vi "Edit_Template_File.vi"(0 "Mode":T2(ring), 7 "Template Filename":path, 11 "Data Filename":path) -> (6 "Template Filename Out":path)   [LabVIEW 2015]
uses:
  Anemometry/Anemometry Sub Vis/Data_plotting_vis/File_Template_Clus.ctl
  Anemometry/Anemometry Sub Vis/Controls/Global_mode.ctl
panel:
  out "index of element":i32
  in  "Add New Channel Named":bool
  in  "Edit Maths Equation":bool
  out "Current Case Name":string
  in  "Organise Channels":bool
  in  "Add New Channels Fr File":bool
  in  "OK":bool
  in  "Search String":string
  in  "Listbox":i32(listbox)
  out "Channel Name":string
  in  "Cluster":T1 {"Tolerance" min=0.0 format="%#.4f"}
  # "> 20  or  <20  or  =hello   or \n£hello  (not equal to hello)"
  # "<<Characters_to_Match>>  <<Replace_Whole_String_with_this>>"
  # "<<Channel_Name>> contains <<Characters to match>> or\n<<Channel_Name>> does not contain <<Characters to match>>"
  # "<<Channel_Name_A>> + <<Channel_Name_B>> or\nConcatenate <<Channel_Name_A>> and <<Channel_Name_B>>"
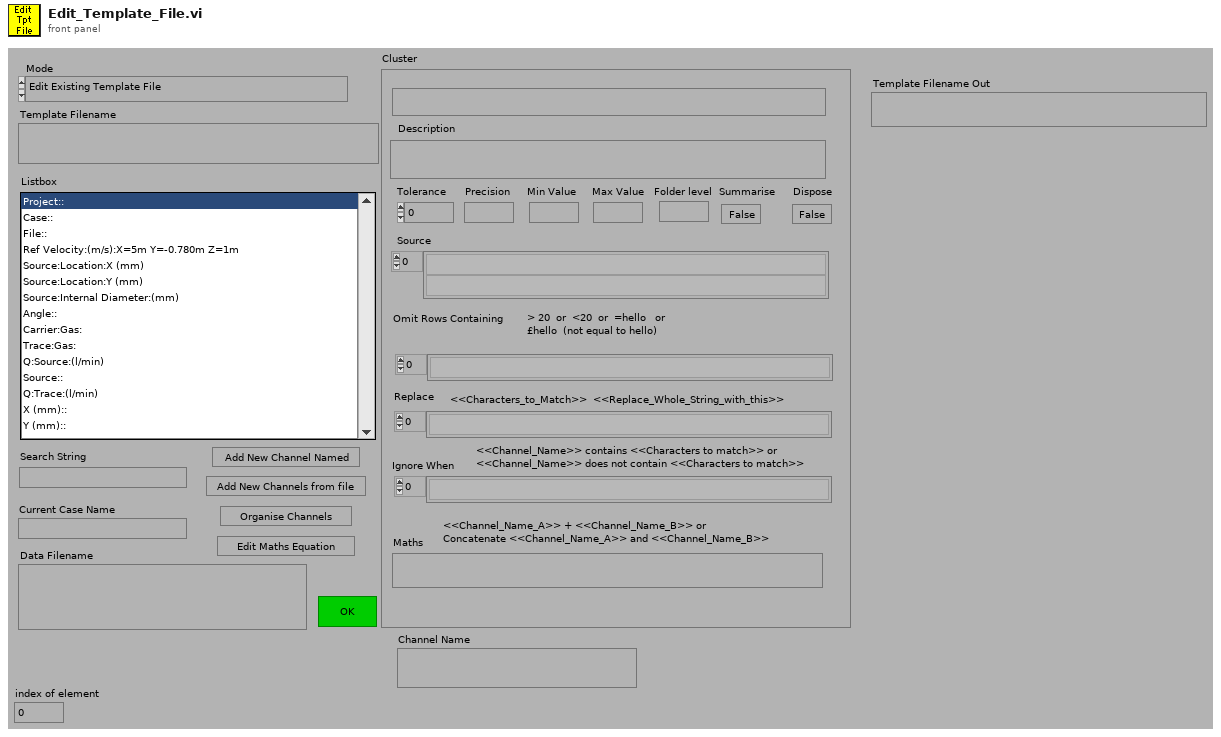
[diagram p1: front panel]
types:
  T1 = typedef "File_Template_Clus.ctl" = cluster{"Template Channel Name":string, "Description":string, "Tolerance":dbl, "Precision":string, "Folder level":string, "Source":string[], "Replace":string[], "Summarise":bool, "Dispose":bool, "Min Value":string, "Maths":string, "Omit Rows Containing":string[], "Ignore When":string[], "Max Value":string}
  T2 = enum16{"Edit Existing Template File", "Create New Template File"}
  T3 = typedef "Global_mode.ctl" = enum16{"Read Global", "Load Global From File", "Write Global to File"}
  T4 = enum16{"Read Channels From File", "Read Channels from Server"}
  T5 = enum32{"existing file", "new file", "new or existing file", "existing dir", "new dir", "new or existing dir", "existing file (use LLBs)", "new file (use LLBs)", "new or existing file (use LLBs)", "new or existing file or directory (use LLBs)"}
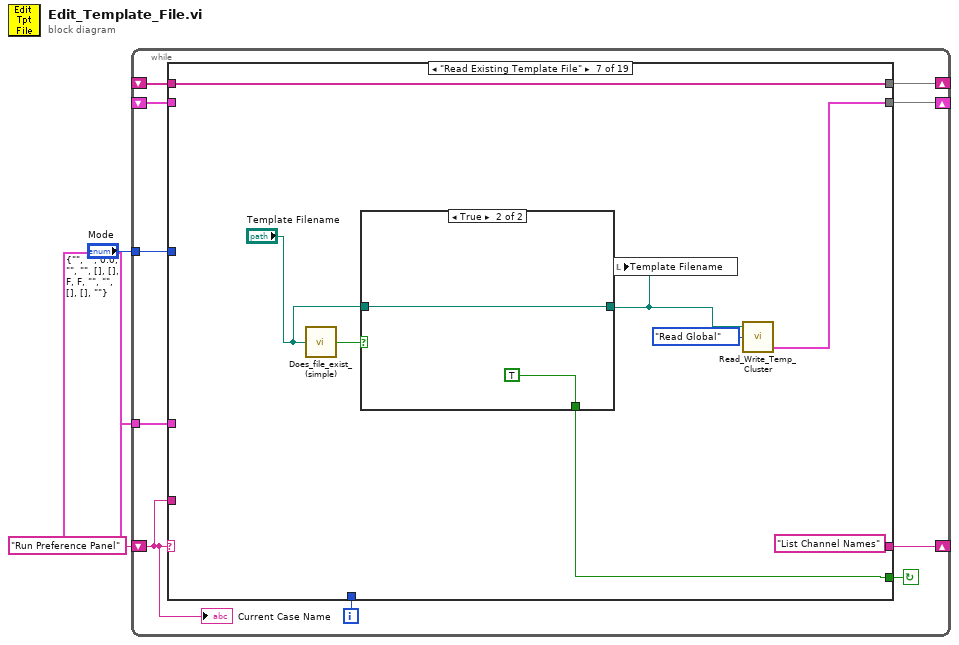
[diagram p0: block diagram]
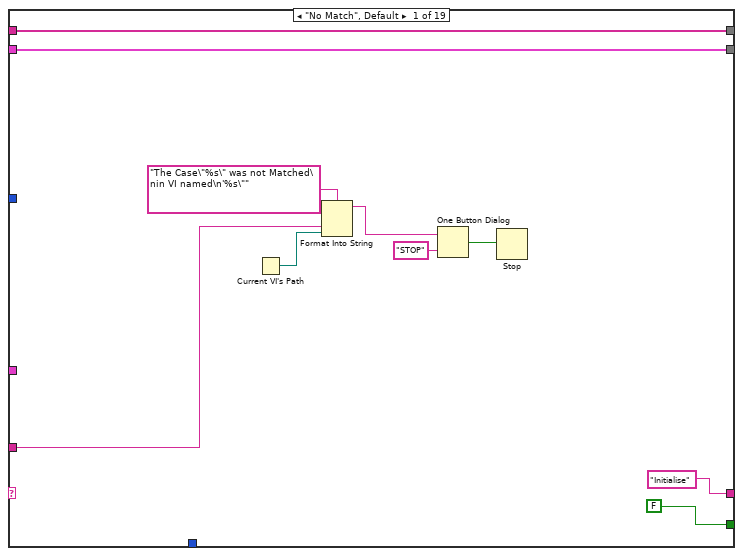
[diagram p2: hidden frame]
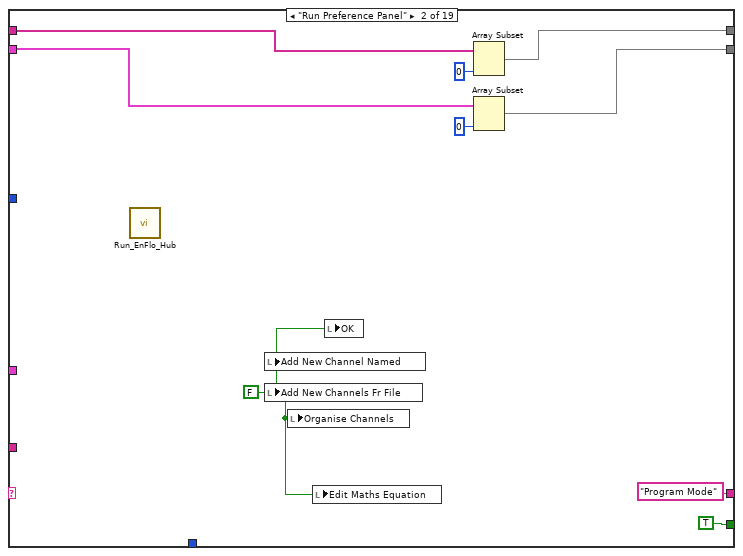
[diagram p3: hidden frame]
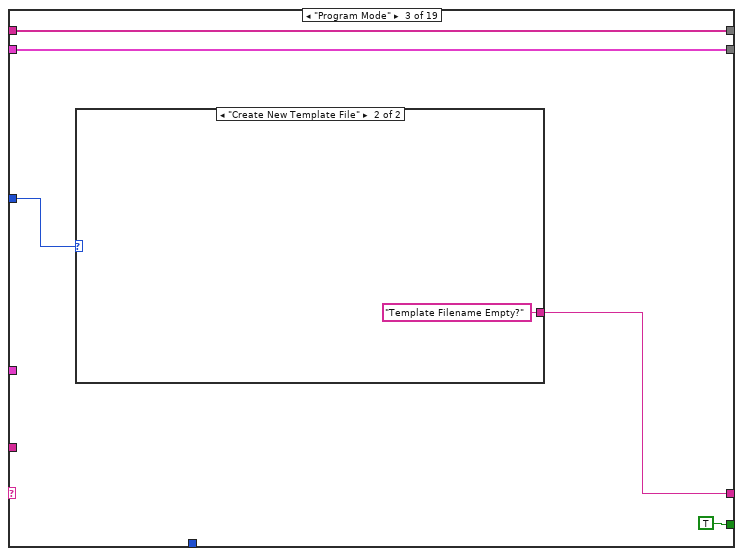
[diagram p4: hidden frame]
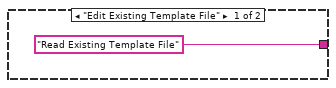
[diagram p5: hidden frame]
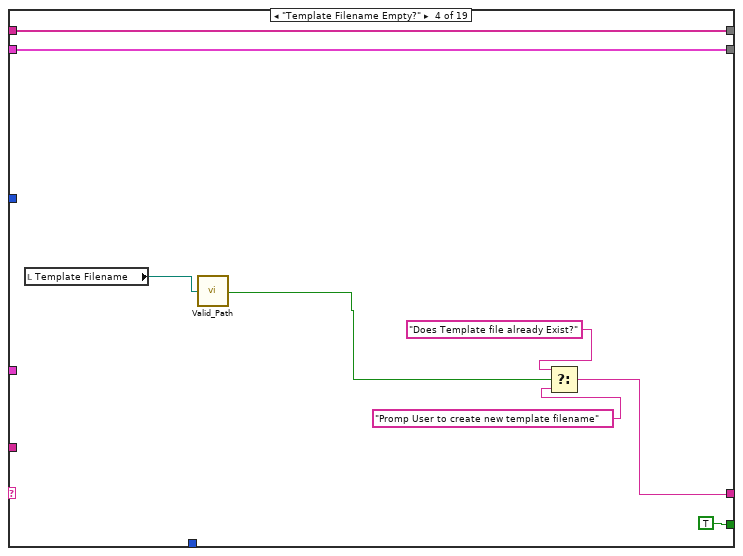
[diagram p6: hidden frame]
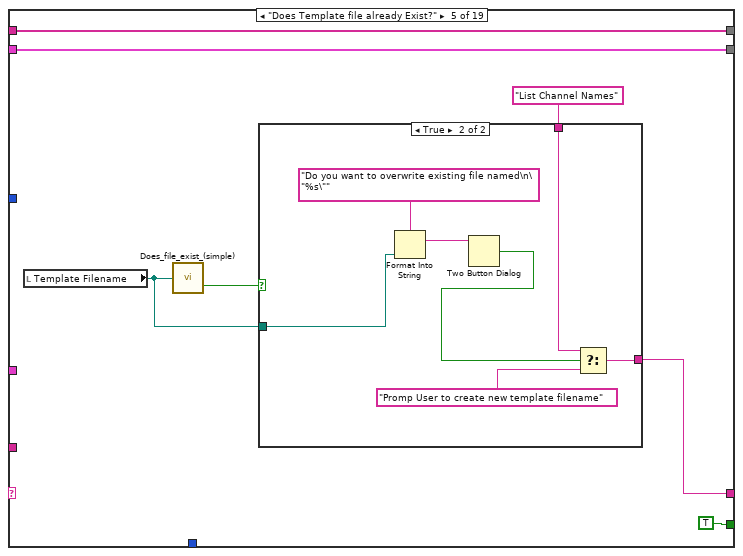
[diagram p7: hidden frame]
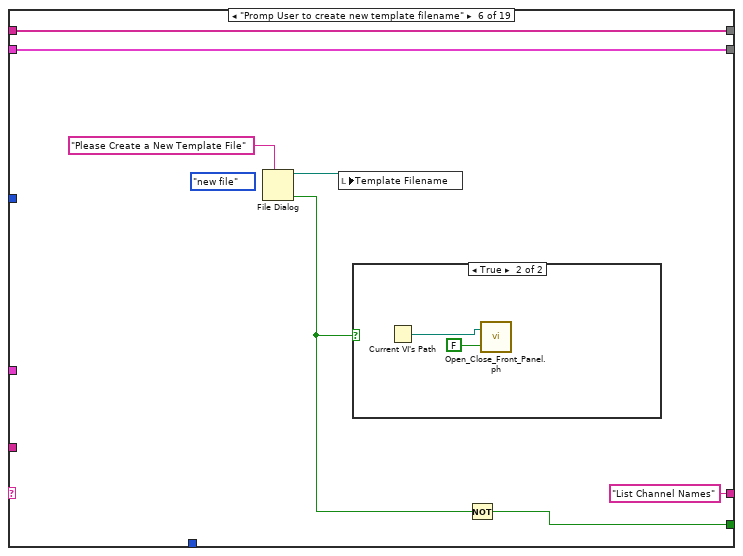
[diagram p9: hidden frame]
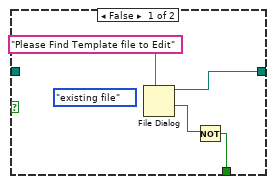
[diagram p11: hidden frame]
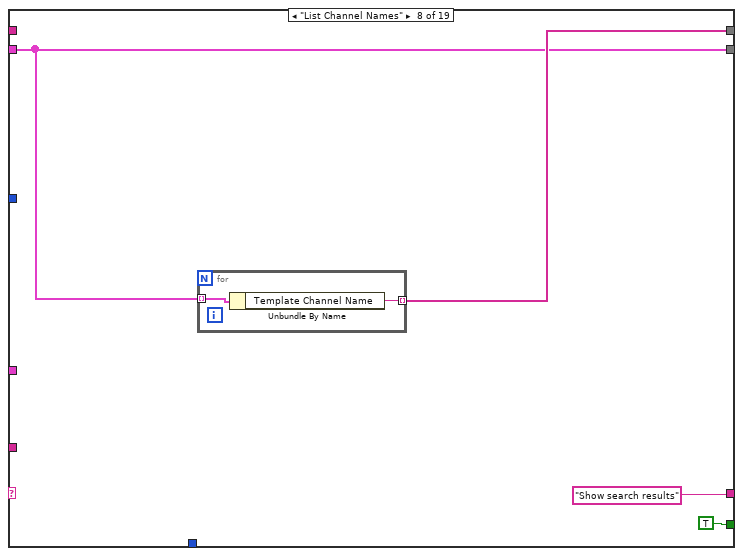
[diagram p12: hidden frame]
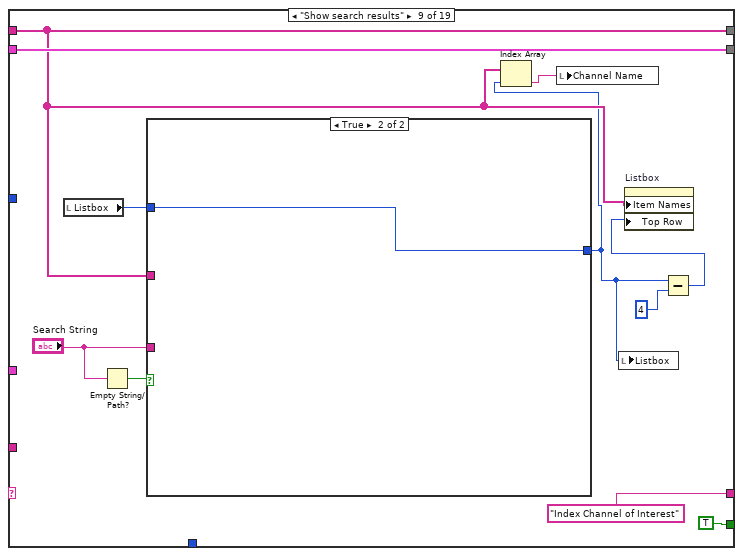
[diagram p13: hidden frame]
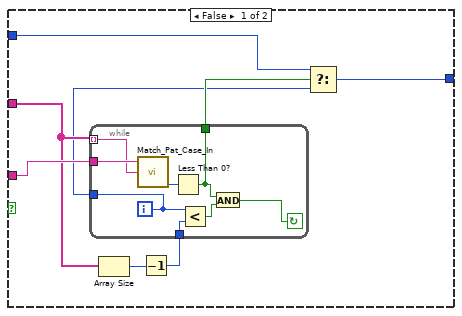
[diagram p14: hidden frame]
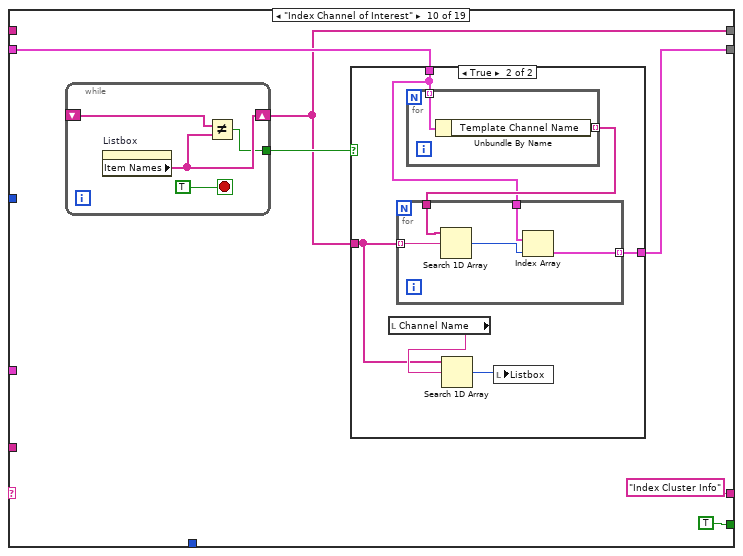
[diagram p15: hidden frame]
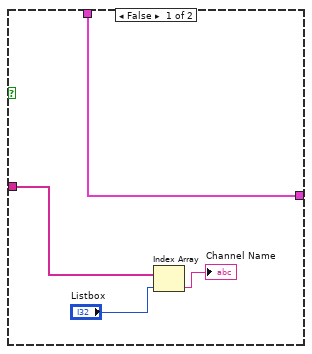
[diagram p16: hidden frame]
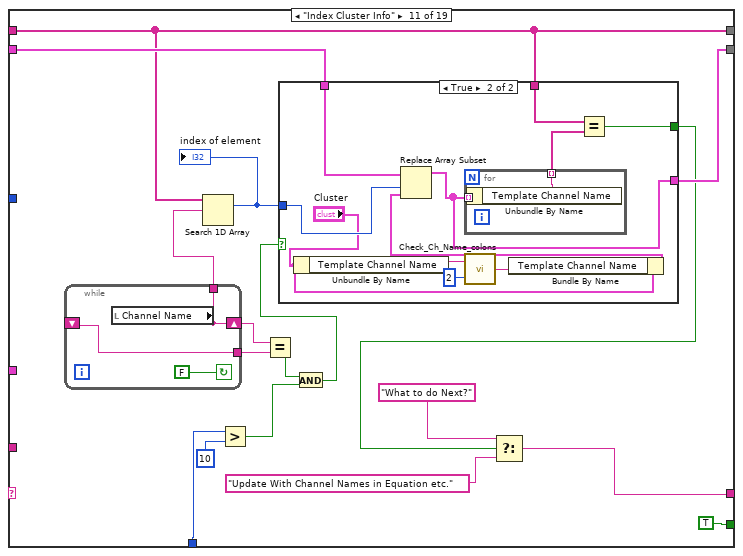
[diagram p17: hidden frame]
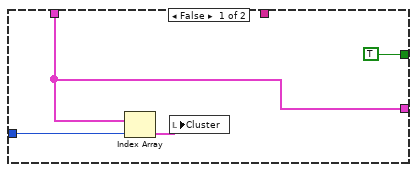
[diagram p18: hidden frame]
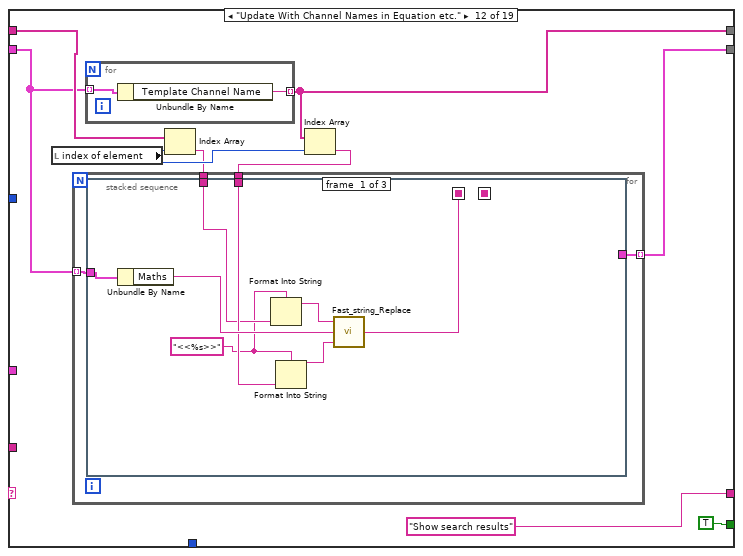
[diagram p19: hidden frame]
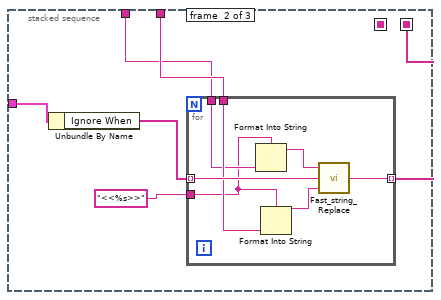
[diagram p20: hidden frame]
diagram:
  n1 = while {
    tunnel: T1 {"Template Channel Name"="", "Description"="", "Tolerance"=0.0, "Precision"="", "Folder level"="", "Source"=[], "Replace"=[], "Summarise"=FALSE, "Dispose"=FALSE, "Min Value"="", "Maths"="", "Omit Rows Containing"=[], "Ignore When"=[], "Max Value"=""} ("Cluster") -> [w6]
    shift-left: _ -> [w7]
    shift-right: [w8] -> _
    tunnel: "Mode" -> [w11]
    shift-left: _ -> [w9]
    shift-right: [w10] -> _
    shift-left: "Run Preference Panel" -> [w5]
    shift-right: [w12] -> _
    i -> [w4]
    stop <- w13 continue-if-true
    n2 = case shown="\"Read Existing Template File\"" w5 {
      tunnel: [FALSE TRUE TRUE TRUE TRUE w64 w72 TRUE TRUE TRUE TRUE TRUE TRUE TRUE TRUE TRUE TRUE TRUE FALSE] -> w13
      tunnel: ["Initialise" "Program Mode" w33 w44 w49 "List Channel Names" ("t") "List Channel Names" "Show search results" "Index Channel of Interest" "Index Cluster Info" w154 "Show search results" "Update cluster info after edit" "Update cluster info after edit" "Update cluster info after edit" "Save Template File" ("t") w332 w342 "End" ("t")] -> w12
      tunnel: w5 -> [w18 _ _ _ _ _ _ _ _ _ _ _ _ _ _ _ _ _ _]
      tunnel: w11 -> [_ _ w36 _ _ _ _ _ _ _ _ _ _ _ _ _ _ _ _]
      tunnel: [w14 w25 w34 w45 w52 w68 w75 w86 w98 w122 w157 w189 w227 w269 w286 w310 w335 w347 w361] -> w10
      tunnel: w9 -> [w14 w26 w34 w45 w52 w68 _ w86 w98 w123 w161 w188 w229 w270 w291 w310 w335 w348 w361]
      tunnel: [w15 w28 w35 w46 w53 w69 w74 w88 w94 w120 w153 w190 w228 w271 w293 w312 w336 w351 w362] -> w8
      tunnel: w7 -> [w15 w29 w35 w46 w53 w69 w74 _ w94 _ w153 w191 w230 w272 w293 w312 w336 w351 w362]
      tunnel: w6 -> [_ _ _ _ _ _ _ _ _ _ _ _ w226 _ _ _ _ _ _]
      tunnel: w4 -> [_ _ _ _ _ _ _ _ _ _ w151 _ _ _ _ _ _ _ _]
      frame "No Match", Default {
        n3 = Current VI's Path() -> (path=w17:path)
        n4 = Format Into String(format string="The Case\"%s\" was not Matched\nin VI named\n'%s\"" ("Format String"), w18, w17) -> (resulting string=w21:string)  [unwired: 2 in, 1 out]
        n5 = One Button Dialog(message=w21, button name ("OK")="STOP") -> (true=w19:bool)
        n6 = Stop(stop? (T)=w19) -> ()
      }
      frame "Run Preference Panel" {
        w24 = FALSE ("Add channel Fr Results File")
        n7 = call "Run_EnFlo_Hub.vi"() -> ()  [unwired: 8 out]
        n8 = local write "Add New Channel Named"(w24) -> ()
        n9 = local write "Add New Channels Fr File"(w24) -> ()
        n10 = local write "Organise Channels"(w24) -> ()
        n11 = local write "Edit Maths Equation"(w24) -> ()
        n12 = local write "OK"(w24) -> ()
        n13 = Array Subset(array=w29, length=0 ("Array Length")) -> (w28:string[])  [unwired: 1 in]
        n14 = Array Subset(array=w26, length=0 ("Array Length")) -> (w25:T1[])  [unwired: 1 in]
      }
      frame "Program Mode" {
        n15 = case shown="\"Create New Template File\"" w36 {
          tunnel: ["Read Existing Template File" "Template Filename Empty?"] -> w33
          frame "Edit Existing Template File" {
          }
          frame "Create New Template File" {
          }
        }
      }
      frame "Template Filename Empty?" {
        n16 = local read "Template Filename"() -> (w43:path)
        n17 = call "Valid_Path.vi"("Filename"=w43) -> ("Valid Path?"=w42:bool)
        n18 = Select(t="Does Template file already Exist?", s=w42, f="Promp User to create new template filename" ("t")) -> (s? t:f=w44:string)
      }
      frame "Does Template file already Exist?" {
        n19 = local read "Template Filename"() -> (w50:path)
        n20 = call "Does_file_exist_(simple).vi"("Pathname"=w50) -> ("exists?"=w51:bool)
        n21 = case shown="True" w51 {
          tunnel: w50 -> [_ w62]
          tunnel: [w55 w57] -> w49
          tunnel: "List Channel Names" ("t") -> [w55 w56]
          frame False {
          }
          frame True {
            n22 = Format Into String(format string="Do you want to overwrite existing file named\n\"%s\"" ("Format String"), w62) -> (resulting string=w60:string)  [unwired: 2 in, 1 out]
            n23 = Two Button Dialog(message=w60) -> (T button?=w58:bool)  [unwired: 2 out]
            n24 = Select(t=w56, s=w58, f="Promp User to create new template filename") -> (s? t:f=w57:string)
          }
        }
      }
      frame "Promp User to create new template filename" {
        (unwired) T5."new file" ("select mode (2)")
        n25 = File Dialog(7:"Please Create a New Template File" ("prompt")) -> (1:w63:bool, 3:w67:path)  [unwired: 1 in, 7 out]
        n26 = local write "Template Filename"(w67) -> ()
        n27 = case shown="True" w63 {
          frame False {
          }
          frame True {
            n28 = Current VI's Path() -> (path=w71:path)
            n29 = call "Open_Close_Front_Panel.ph.vi"("Front Panel Window:Open"=FALSE, "VI path"=w71) -> ()  [unwired: 2 out]
          }
        }
        n30 = Not(x=w63) -> (.not. x?=w64:bool)
      }
      frame "Read Existing Template File" {
        n31 = call "Does_file_exist_(simple).vi"("Pathname"="Template Filename") -> ("exists?"=w78:bool)
        n32 = case shown="True" w78 {
          tunnel: [w83 w85] -> w73
          tunnel: "Template Filename" -> [_ w85]
          tunnel: [w80 TRUE] -> w72
          frame False {
            (unwired) T5."existing file" ("select mode (2)")
            n33 = File Dialog(7:"Please Find Template file to Edit" ("prompt")) -> (1:w81:bool, 3:w83:path)  [unwired: 1 in, 7 out]
            n34 = Not(x=w81) -> (.not. x?=w80:bool)
          }
          frame True {
          }
        }
        n35 = local write "Template Filename"(w73) -> ()
        n36 = call "Read_Write_Temp_Cluster.vi"("Mode"=Global_mode."Read Global", "Template File"=w73) -> ("Template Info Array Out"=w75:T1[])  [unwired: 1 in, 2 out]
      }
      frame "List Channel Names" {
        n37 = for {
          tunnel: w86 -> [w91] mode=indexing
          tunnel: [w90] -> w88 mode=indexing
          n38 = Unbundle By Name(w91) -> ("Template Channel Name"=w90:string)
        }
      }
      frame "Show search results" {
        n39 = local read "Listbox"() -> (w93:i32)
        n40 = Empty String/Path?(string/path="Search String") -> (empty?=w100:bool)
        n41 = case shown="True" w100 {
          tunnel: "Search String" -> [w110 _]
          tunnel: w94 -> [w109 _]
          tunnel: w93 -> [w105 w119]
          tunnel: [w103 w119] -> w92
          frame False {
            n42 = Array Size(array=w109) -> (size(s)=w108:i32)
            n43 = Decrement(x=w108) -> (x-1=w107:i32)
            n44 = while {
              tunnel: w110 -> [w118]
              tunnel: w109 -> [w117] mode=indexing
              tunnel: w107 -> [w115]
              tunnel: [w112] -> w106
              tunnel: [w111] -> w104
              i -> [w111]
              stop <- w113 continue-if-true
              n45 = call "Match_Pat_Case_In.vi"("String to match"=w118, "String"=w117) -> ("offset past match"=w116:i32)  [unwired: 1 in, 3 out]
              n46 = Less Than 0?(x=w116) -> (x < 0?=w112:bool)
              n47 = Less?(x=w111, y=w115) -> (x < y?=w114:bool)
              n48 = And(x=w112, y=w114) -> (x .and. y?=w113:bool)
            }
            n49 = Select(t=w105, s=w106, f=w104) -> (s? t:f=w103:i32)
          }
          frame True {
          }
        }
        n50 = Index Array(array=w94, index=w92) -> (element=w95:string)
        n51 = local write "Channel Name"(w95) -> ()
        n52 = local write "Listbox"(w92) -> ()
        n53 = Subtract(x=w92, y=4) -> (x-y=w96:i32)
        n54 = property on="Listbox" class="LstBox (strict)"("Item Names"=w94, "Top Row"=w96) -> ()  [unwired: 2 in, 2 out]
      }
      frame "Index Channel of Interest" {
        n55 = while {
          shift-right: [w145] -> w120
          shift-left: _ -> [w146]
          tunnel: [w143] -> w121
          stop <- TRUE stop-if-true
          n56 = property on="Listbox" class="LstBox (strict)"() -> ("Item Names"=w145:string[])  [unwired: 2 in, 2 out]
          n57 = Not Equal?(x=w146, y=w145) -> (x != y?=w143:bool)
        }
        n58 = case shown="True" w121 {
          tunnel: w120 -> [w127 w131]
          tunnel: w123 -> [w129 w134]
          tunnel: [w129 w133] -> w122
          frame False {
            n59 = Index Array(array=w127, index="Listbox") -> (element=→"Channel Name":string)
          }
          frame True {
            n60 = local read "Channel Name"() -> (w132:string)
            n61 = for {
              tunnel: w134 -> [w142] mode=indexing
              tunnel: [w141] -> w135 mode=indexing
              n62 = Unbundle By Name(w142) -> ("Template Channel Name"=w141:string)
            }
            n63 = for {
              tunnel: w135 -> [w140]
              tunnel: w131 -> [w139] mode=indexing
              tunnel: w134 -> [w137]
              tunnel: [w136] -> w133 mode=indexing
              n64 = Search 1D Array(1D array=w140, element=w139) -> (index of element=w138:i32)  [unwired: 1 out]
              n65 = Index Array(array=w137, index=w138) -> (element=w136:T1)
            }
            n66 = Search 1D Array(1D array=w131, element=w132) -> (index of element=w130:i32)  [unwired: 1 out]
            n67 = local write "Listbox"(w130) -> ()
          }
        }
      }
      frame "Index Cluster Info" {
        n68 = while {
          tunnel: [w165] -> w158
          tunnel: [w166] -> w159
          shift-left: _ -> [w166]
          shift-right: [w165] -> w160
          stop <- FALSE continue-if-true
          n69 = local read "Channel Name"() -> (w165:string)
        }
        n70 = Search 1D Array(1D array=w153, element=w158) -> (index of element=w162:i32)  [unwired: 1 out]
        "index of element" <- w162
        n71 = Greater?(x=w151, y=10) -> (0:w148:bool)
        n72 = Equal?(x=w160, y=w159) -> (x = y?=w149:bool)
        n73 = And(x=w149, y=w148) -> (x .and. y?=w147:bool)
        n74 = case shown="True" w147 {
          tunnel: w162 -> [w170 w180]
          tunnel: w161 -> [w168 w181]
          tunnel: [w168 w177] -> w157
          tunnel: w153 -> [_ w178]
          tunnel: [TRUE w176] -> w152
          frame False {
            n75 = Index Array(array=w168, index=w170) -> (element=w169:T1)
            n76 = local write "Cluster"(w169) -> ()
          }
          frame True {
            n77 = Unbundle By Name("Cluster") -> ("Template Channel Name"=w174:string)
            n78 = call "Check_Ch_Name_colons.vi"("No of Colons"=2, "Ch Name in"=w174) -> ("Ch Name out"=w173:string)
            n79 = Bundle By Name(cluster="Cluster", "Template Channel Name"=w173) -> (w171:T1)
            n80 = Replace Array Subset(array=w181, new element=w171, index=w180) -> (w177:T1[])
            n81 = for {
              tunnel: w177 -> [w183] mode=indexing
              tunnel: [w182] -> w179 mode=indexing
              n82 = Unbundle By Name(w183) -> ("Template Channel Name"=w182:string)
            }
            n83 = Equal?(x=w178, y=w179) -> (x = y?=w176:bool)
          }
        }
        n84 = Select(t="What to do Next?", s=w152, f="Update With Channel Names in Equation etc.") -> (s? t:f=w154:string)
      }
      frame "Update With Channel Names in Equation etc." {
        n85 = local read "index of element"() -> (w186:i32)
        n86 = for {
          tunnel: w188 -> [w223] mode=indexing
          tunnel: [w222] -> w190 mode=indexing
          n87 = Unbundle By Name(w223) -> ("Template Channel Name"=w222:string)
        }
        n88 = Index Array(array=w191, index=w186) -> (element=w185:string)
        n89 = Index Array(array=w190, index=w186) -> (element=w184:string)
        n90 = for {
          tunnel: w188 -> [w194] mode=indexing
          tunnel: w184 -> [w196]
          tunnel: [w193] -> w189 mode=indexing
          tunnel: w185 -> [w195]
          n91 = stacked-sequence {
            seq-local: [w198 _ _] -> [_ _ w221]
            seq-local: [_ w206 _] -> [_ _ w219]
            tunnel: w194 -> [w204 w210 w218]
            tunnel: w196 -> [w202 w208 _]
            tunnel: w195 -> [w199 w207 _]
            tunnel: [_ _ w220] -> w193
            frame #0 {
              w197 = "<<%s>>" ("Format String")
              n92 = Unbundle By Name(w204) -> ("Maths"=w203:string)
              n93 = Format Into String(format string=w197, w199) -> (resulting string=w200:string)  [unwired: 2 in, 1 out]
              n94 = Format Into String(format string=w197, w202) -> (resulting string=w201:string)  [unwired: 2 in, 1 out]
              n95 = call "Fast_string_Replace.vi"("Replace match with:"=w201, "Input String"=w203, "regular expression"=w200) -> ("Output String"=w198:string)  [unwired: 2 out]
            }
            frame #1 {
              n96 = Unbundle By Name(w210) -> ("Ignore When"=w209:string[])
              n97 = for {
                tunnel: w209 -> [w217] mode=indexing
                tunnel: w208 -> [w216]
                tunnel: w207 -> [w213]
                tunnel: [w212] -> w206 mode=indexing
                tunnel: "<<%s>>" ("Format String") -> [w211]
                n98 = Format Into String(format string=w211, w213) -> (resulting string=w214:string)  [unwired: 2 in, 1 out]
                n99 = Format Into String(format string=w211, w216) -> (resulting string=w215:string)  [unwired: 2 in, 1 out]
                n100 = call "Fast_string_Replace.vi"("Replace match with:"=w215, "Input String"=w217, "regular expression"=w214) -> ("Output String"=w212:string)  [unwired: 2 out]
              }
            }
            frame #2 {
              n101 = Bundle By Name(cluster=w218, "Maths"=w221, "Ignore When"=w219) -> (w220:T1)
            }
          }
        }
      }
      frame "Select New Channel" {
        n102 = local read "Add New Channel Named"() -> (w225:bool)
        n103 = case shown="True" w225 {
          tunnel: [w235 w241] -> w231
          tunnel: [FALSE ("Add channel Fr Results File") FALSE ("Add channel Fr Results File")] -> w224
          frame False {
            n104 = call "Select_a_Channel.vi"("Mode"=T4."Read Channels From File", "Data Filename"="Data Filename") -> ("Selected Channel Names"=w235:string[], "Data Filename Out"=w237:path)  [unwired: 1 in, 4 out]
            n105 = local write "Data Filename"(w237) -> ()
          }
          frame True {
            n106 = call "Input_String_Dialog.vi"("Message to user"="Enter New Channel Name") -> ("Ok Out"=w243:bool, "Output string"=w244:string)  [unwired: 1 in]
            n107 = Build Array(w244) -> (w242:string[])
            n108 = Select(t=w242, s=w243, f=string[] []) -> (s? t:f=w241:string[])
          }
        }
        n109 = for {
          tunnel: w231 -> [w250] mode=indexing
          shift-right: [w248] -> w228
          shift-left: w230 -> [w249]
          shift-right: [w251] -> w227
          shift-left: w229 -> [w252]
          tunnel: w226 -> [w254]
          n110 = Build Array(w250) -> (w257:string[])
          n111 = while {
            tunnel: [w258] -> w247
            tunnel: w250 -> [w260]
            tunnel: w249 -> [w261]
            i -> [w259]
            stop <- w262 continue-if-true
            n112 = case shown="1, Default" w259 {
              tunnel: w259 -> [_ w265]
              tunnel: [w264 w267] -> w258
              tunnel: w260 -> [w264 w266]
              frame 0 {
              }
              frame 1, Default {
                n113 = Format Into String(format string="%s_DUPLICATE%d" ("Format String"), w266, w265) -> (resulting string=w267:string)  [unwired: 2 in, 1 out]
              }
            }
            n114 = Search 1D Array(1D array=w261, element=w258) -> (index of element=w263:i32)  [unwired: 1 out]
            n115 = Greater Or Equal To 0?(x=w263) -> (x >= 0?=w262:bool)
          }
          n116 = Bundle By Name(cluster=w254, "Template Channel Name"=w247, "Source"=w257, "Summarise"=TRUE ("Bundle Element"), "Dispose"=FALSE ("Bundle Element"), "Tolerance"=1.0 ("Bundle Element")) -> (w253:T1)
          n117 = Build Array (concatenate)(w252, w253) -> (w251:T1[])
          n118 = Build Array (concatenate)(w249, w247) -> (w248:string[])
        }
        n119 = local write "Add New Channel Named"(w224) -> ()
        n120 = local write "Add New Channels Fr File"(w224) -> ()
      }
      frame "Organise Channels" {
        n121 = call "Organise_String_Array.vi"("Input Array"=w272) -> ("Output Array"=w271:string[])
        n122 = for {
          tunnel: w272 -> [w280]
          tunnel: w271 -> [w279] mode=indexing
          tunnel: w270 -> [w277]
          tunnel: [w276] -> w269 mode=indexing
          n123 = Search 1D Array(1D array=w280, element=w279) -> (index of element=w278:i32)  [unwired: 1 out]
          n124 = Index Array(array=w277, index=w278) -> (element=w276:T1)
        }
        n125 = local write "Organise Channels"(FALSE ("Add channel Fr Results File")) -> ()
      }
      frame "Edit Maths Equation" {
        n126 = local write "Edit Maths Equation"(FALSE ("Add channel Fr Results File")) -> ()
        n127 = property on="Listbox" class="LstBox (strict)"() -> ("Item Names"=w283:string[])  [unwired: 2 in, 2 out]
        n128 = local read "Listbox"() -> (w294:i32)
        n129 = Index Array(array=w283, index=w294) -> (element=w292:string)
        n130 = Search 1D Array(1D array=w293, element=w292) -> (index of element=w288:i32)  [unwired: 1 out]
        n131 = Index Array(array=w291, index=w288) -> (element=w287:T1)
        n132 = Unbundle By Name(w287) -> ("Template Channel Name"=w290:string, "Maths"=w289:string)
        n133 = call "Edit_Maths_Equation.vi"("Template Info Array"=w291, "Maths Equation In"=w289, "Channel Name"=w290) -> ("Template Info Array Out"=w285:T1[], "Maths Equation Out"=w282:string)  [unwired: 1 out]
        n134 = Empty String/Path?(string/path=w282) -> (empty?=w281:bool)
        n135 = case shown="False" w281 {
          tunnel: w283 -> [w299 _]
          tunnel: w282 -> [w298 _]
          frame False {
            w300 = TRUE  # Dialog Box (T)
            n136 = call "Do_channel_maths.vi"("Channel Names"=w299, "Maths Equation"=w298) -> ("Error String"=w304:string)  [unwired: 2 in, 3 out]
            n137 = Empty String/Path?(string/path=w304) -> (empty?=w306:bool)
            n138 = Not(x=w306) -> (.not. x?=w303:bool)
            n139 = Bundle By Name(cluster=errorcluster {"status"=FALSE, "code"=0, "source"=""} ("error in (no error)"), "source"=w304, "status"=w303) -> (w302:errorcluster)
            n140 = call "EnFlo_Error_Handler.vi"("error in (no error)"=w302, "Error Type"="Maths Equation", "Dialog Box (T)"=w300) -> ()  [unwired: 3 out]
          }
          frame True {
          }
        }
        n141 = Bundle By Name(cluster=w287, "Maths"=w282) -> (w284:T1)
        n142 = Replace Array Subset(array=w285, new element=w284, index=w288) -> (w286:T1[])
      }
      frame "Update cluster info after edit" {
        n143 = local read "Channel Name"() -> (w308:string)
        n144 = Search 1D Array(1D array=w312, element=w308) -> (index of element=w311:i32)  [unwired: 1 out]
        n145 = Index Array(array=w310, index=w311) -> (element=w309:T1)
        n146 = local write "Cluster"(w309) -> ()
      }
      frame "What to do Next?" {
        n147 = while {
          tunnel: [w339] -> w330
          shift-left: _ -> [w339]
          shift-right: [w340] -> w331
          stop <- FALSE continue-if-true
          n148 = local read "Search String"() -> (w340:string)
        }
        n149 = Not Equal?(x=w331, y=w330) -> (x != y?=w327:bool)
        n150 = Select(t="List Channel Names", s=w327, f="Index Channel of Interest") -> (s? t:f=w324:string)
        n151 = Select(t="Select New Channel", s="Add New Channels Fr File", f=w324) -> (s? t:f=w321:string)
        n152 = Select(t="Organise Channels", s="Organise Channels", f=w321) -> (s? t:f=w314:string)
        n153 = Select(t="Edit Maths Equation", s="Edit Maths Equation", f=w314) -> (s? t:f=w316:string)
        n154 = Select(t="Select New Channel", s="Add New Channel Named", f=w316) -> (s? t:f=w315:string)
        n155 = Select(t="Save Template File", s="OK", f=w315) -> (s? t:f=w332:string)
      }
      frame "Save Template File" {
        n156 = for {
          tunnel: w348 -> [w353] mode=indexing
          tunnel: [w352] -> w347 mode=indexing
          n157 = Unbundle By Name(w353) -> ("Template Channel Name"=w355:string)
          n158 = call "Check_Ch_Name_colons.vi"("No of Colons"=2, "Ch Name in"=w355) -> ("Ch Name out"=w354:string)
          n159 = Bundle By Name(cluster=w353, "Template Channel Name"=w354) -> (w352:T1)
        }
        n160 = local write "Mode"(T2."Edit Existing Template File" ("Mode")) -> ()
        n161 = local read "Template Filename"() -> (w346:path)
        "Template Filename Out" <- w346
        n162 = local read "OK"() -> (w345:bool)
        n163 = call "Read_Write_Temp_Cluster.vi"("Template Info Array"=w347, "Mode"=Global_mode."Write Global to File", "Template File"=w346) -> ()  [unwired: 3 out]
        n164 = Select(t="Close Panel", s=w345, f="List Channel Names") -> (s? t:f=w342:string)
      }
      frame "Close Panel" {
        n165 = Current VI's Path() -> (path=w358:path)
        n166 = call "Open_Close_Front_Panel.ph.vi"("Front Panel Window:Open"=FALSE, "VI path"=w358) -> ()  [unwired: 2 out]
      }
    }
    "Current Case Name" <- w5
  }
